vi "LCSS classification.vi"(9 "cluster centers":string[](array[string])=["1 0 -1 1 -1 0 -4 1 -4 0 1", "2 0 -1 2 -1 0 -2 2 -2 0 2", "3 0 -3 3 -3 0 -2 3 -2 0 3", "4 0 -3 4 -3 0 -4 4 -4 0 4", "-1 1 -4 0 -4 4 -3 4 -4 0 -4 1 -1", "-1 2 -2 0 -2 3 -3 3 -2 0 -2 2 -1", "-4 1 -1 0 -1 2 -2 2 -1 0 -1 1 -4", "-4 4 -3 0 -3 3 -2 3 -3 0 -3 4 -4", "0 -4 1 -1 0 -3 3 -2 3 -3 0 -1 1 -4 0", "0 -4 4 -3 0 -1 2 -2 2 -1 0 -3 4 -4 0"], 11 "Patterns in":string[](array[string])=["0 4 0", "4 0 4", "0 4 0", "4 0 4", "0 4 0", "4 0 4", "0 4 0", "4 0 -2", "0 -2 3", "-2 3 0", "3 0 3", "0 3 0", "3 0 4", "0 4 0", "-2 0 1", "0 1 0", "1 0 -4", "0 -4 4", "-2 2 0", "2 0 -1", "0 -1 -4", "-1 -4 1", "-4 1 0", "1 0 3", "0 3 0", "-1 0 -1", "0 -1 2", "0 -1 1", "-1 1 0", "1 0 4", "0 4 0", "4 0 3", "0 3 -2", "3 -2 0", "-2 0 -2", "0 -2 3", "-2 3 -2", "3 -2 0", "-2 0 4", "0 4 0", "4 0 -2", "0 -2 2", "2 -1 0", "-1 0 4", "0 4 0", "4 0 2", "0 2 0", "2 0 -2", "0 -2 0", "1 -1 0", "-1 0 3", "0 3 0", "3 0 -4", "0 -4 4", "-4 4 -4", "4 -4 0", "2 -1 0", "-1 0 3", "0 3 -2", "3 -2 0", "-2 0 -3", "0 -3 0", "-3 0 3", "0 3 0", "3 0 -3", "0 -3 0", "0 4 0", "4 0 4", "0 4 -4", "4 -4 1", "-4 1 -1", "1 -1 0", "-1 0 -3", "0 -3 0", "-3 0 1", "0 1 -4", "1 -4 1", "-4 1 0", "1 0 4", "0 4 0", "4 0 -4", "0 -4 0", "-4 0 -4", "0 -4 4", "-4 4 -4", "4 -4 1", "0 -4 1", "-4 1 0", "1 0 -4", "0 -4 4", "0 4 0", "4 0 -2", "0 -2 2", "-2 2 -2", "2 -2 2", "-2 2 -2", "2 -2 2", "-2 2 -1", "2 -1 0", "-1 0 4", "0 4 0", "4 0 2", "0 2 0", "2 0 4", "0 4 0", "4 0 2", "0 2 -2", "2 -2 0", "-2 0 4", "1 0 -1", "0 -1 0", "-1 0 -1", "0 -1 0", "-1 0 1", "0 1 -1", "-2 2 -2", "2 -2 3", "1 0 -1", "0 -1 0", "-1 0 -1", "0 -1 2", "-1 2 0", "2 0 2", "0 2 -2", "2 -2 0", "-2 0 -4", "0 -4 0", "-2 2 0", "2 0 3", "0 3 -2", "3 -2 2", "1 -1 0", "-1 0 3", "0 4 0", "-2 0 1", "0 1 -4", "1 -4 0", "-4 0 -3", "0 -3 0", "1 0 -1", "0 -1 2", "-1 2 -1", "2 -1 1", "-1 1 -4", "-2 0 -1", "0 -1 1", "0 3 0", "3 0 3", "0 3 0", "3 0 3", "0 3 -2", "-4 0 -4", "0 -4 4", "0 4 0", "4 0 -4", "0 -4 0", "-4 0 -4", "-2 2 0", "2 0 4", "0 4 -4", "4 -4 0", "-4 0 2", "0 2 -2"]) -> (0 "Assigned cluster (0) unassigned":string[](array[string]), 1 "patterns in, distance values":string[][](array[string]), 2 "Assigned cluster 2nd method":string[](array[string]), 3 "Cluster element count":i32[](array[numeric]), 4 "Assigned cluster 3rd method 2":string[](array[string]))   [LabVIEW 2014]
panel:
  in  "Patterns in 2":string[](array[string])
  out "Array":i32[](array[numeric])
  in  "cluster centers 3":string[](array[string])=["0 1 0 -1 1 0 1 -1 0 -4 1 0 1 -4 0", "0 2 0 -1 2 0 2 -1 0 -2 2 0 2 -2 0", "0 3 0 -3 3 0 3 -3 0 -2 3 0 3 -2 0", "0 4 0 -3 4 0 4 -3 0 -4 4 0 4 -4 0", "-1 1 -4 0 -4 4 -3 4 -4 0 -4 1 -1", "-1 2 -2 0 -2 3 -3 3 -2 0 -2 2 -1", "-4 1 -1 0 -1 2 -2 2 -1 0 -1 1 -4", "-4 4 -3 0 -3 3 -2 3 -3 0 -3 4 -4", "0 -4 1 -1 0 -3 3 -2 3 -3 0 -1 1 -4 0", "0 -4 4 -3 0 -1 2 -2 2 -1 0 -3 4 -4 0"]
  out "x .and. y? 2":bool
  out "x .and. y?":bool
  out "number of elements":i32[](array[numeric])
  in  "LEfty CSS":string[](array[string])=["0 4 0", "0 -2 0", "1 -1 0", "-1 2 -1", "0 2 0", "2 -1 0", "0 3 0", "0 -1 0", "-2 0 3", "0 -4 0", "3 -2 0", "0 3 -2", "0 -3 0", "-1 0 3", "0 -2 0 3", "0 1 -1 0", "0 3 -2 0", "1 -4 0", "-1 0 2", "0 -1 2", "2 0 3", "0 -3 3", "3 -3 0", "3 0 -1 0", "-2 0 -2", "2 -2 0", "-3 3 0", "0 2 0 3", "0 1 0", "0 -2 2", "-4 0 -1", "0 -1 2 -1", "-1 0 -1", "2 -1 2", "-1 3 -2", "3 0 -4", "3 -2 2", "-1 1 -1 0", "-1 2 -1 0", "0 1 -4", "4 -4 0", "2 -3 0", "0 3 0 -2", "2 0 3 0", "0 1 0 -3", "1 0 -3", "-1 0 -4 0", "-4 0 1", "2 0 -2 0", "-1 0 -3", "0 -3 4", "4 0 1", "0 1 -4 0", "0 -1 0 3", "0 -3 3 0", "0 3 -3 0", "0 4 0 2", "0 2 -2 0", "-2 0 -3", "3 0 3", "-1 0 -2", "-2 0 3 0", "2 0 4 0", "0 4 0 -2 3", "0 -3 0 -2", "-3 0 -2 2", "1 0 4 0", "-3 0 2", "0 -2 0 3 -2 0", "1 0 -3 0", "-3 0 -2", "-2 0 -2 0", "0 4 -4", "-1 -3 0", "-2 2 -1", "2 0 -3", "-1 1 0", "2 -1 1", "-2 2 0", "0 -4 0 -1", "0 -1 3 -2 2", "-1 2 -1 2", "-1 2 0", "-1 3 0 -1 0", "2 0 2", "-1 0 2 -3 0", "-1 0 2 0", "-1 4 -4 1", "-1 0 4", "2 -1 0 -1", "2 -1 0 2", "-4 1 -1", "3 0 -4 1", "1 -1 -3 3", "0 3 0", "0 2 0", "0 4 0", "0 -3 4", "0 1 0", "2 -1 0", "0 -1 0", "0 -3 3", "2 0 3", "0 4 -4", "1 -1 0", "0 3 -2", "3 0 3", "0 2 -1", "-4 0 -3", "0 -3 0", "-1 0 4", "-1 0 2", "4 -4 1", "4 -4 0", "0 -2 3", "3 -3 0", "0 1 -1", "0 1 -4 0", "3 0 3 0", "1 -4 0", "0 2 0 3", "3 -2 0", "0 3 0 3", "-1 0 3", "1 -1 0 4", "0 2 -1 0", "0 -3 4 -4", "3 0 1", "0 -2 0", "0 4 -4 0", "0 3 0 3 0", "1 0 3 0", "3 -2 2", "-4 0 -3 3", "3 0 -3", "0 -3 3 -3 0", "3 0 -2", "-4 1 0", "0 -4 4", "2 -1 0 -3", "0 3 0 1", "2 0 -3", "-3 0 1", "-4 1 -1", "0 2 -2", "-2 3 0", "1 0 1", "0 -1 0 2", "0 3 -2 2", "0 1 0 3", "0 -4 1", "0 -3 3 0", "-2 2 0", "-2 0 3", "1 0 4 0", "4 -4 1 0", "0 1 -1 2", "1 0 1 0", "0 1 0 1", "-1 0 4 -4", "2 -1 0 3", "1 -1 2", "-1 2 -1 0", "0 4 -4 1 -1", "0 -3 4 -4 1", "4 -4 0 -3 3", "0 -4 4 -4", "-1 0 2 -1", "-2 0 -1", "1 -1 0 4 -4", "0 4 0 3", "2 0 4", "4 -4 0 -3", "0 3 0 -2", "0 -3 4 0", "1 0 3", "-4 0 3", "-3 0 2", "0 3 -2 3", "0 2 0 3 0", "0 4 0 2", "4 -3 0", "-3 0 1 0", "0 2 0 -3", "0 1 0 3 0", "0 -4 0", "0 -4 0 -3", "2 -2 0", "2 0 -2", "0 3 -3", "2 -1 0 -3 4", "-1 0 -2", "1 -1 0 3", "-1 0 3 0", "0 -1 2", "0 -3 4 -4 1 0", "0 4 0 -1", "1 0 -3", "0 3 -2 0", "0 1 0 4 0", "0 4 0 -4", "0 4 0 3 -2", "3 -2 0 1 0", "2 -1 0 -3 0", "-3 0 -4", "0 4 -4 1 -1 0", "-1 0 4 -4 0", "0 4 -4 0 2", "-3 0 -1", "0 3 0 1 -1", "-1 0 4 0", "0 1 -1 2 -1 0", "2 -1 0 2", "0 2 0 -1", "-1 0 -1 0", "-1 0 2 -1 0", "0 1 0 2", "0 2 0 -3 4 -4", "1 0 3 0 2", "0 -2 3 -2", "3 -2 0 -1", "0 4 -4 0 -3", "1 0 -4", "-4 0 -3 3 -3 0", "-2 3 -2 0", "-2 3 -2", "0 4 0 2 0", "-4 0 3 0", "0 1 -4", "0 -3 3 0 -2", "0 -2 0 2", "-2 0 2 0", "3 0 -2 0", "-4 0 -3 0", "0 -3 0 3", "0 3 -3 0", "0 -3 4 -3 0 1 0", "0 3 -2 2 0", "2 0 2", "0 2 0 2 0", "0 3 0 -3", "3 0 -3 4", "0 1 0 1 0", "0 -3 3 -2 0 3", "0 -3 4 -4 0 -3 3 -2", "0 -3 0 2 0", "0 2 -2 0", "0 -3 3 -2", "2 0 -4 0 -3 3", "3 0 -2 3", "0 2 0 -2", "0 2 0 4 0", "-2 0 -2 3 0", "0 1 0 3 0 -2", "-3 3 -3", "0 -3 3 -3", "-3 3 -3 0", "1 0 4", "-4 0 2", "-1 0 -1", "3 0 2", "-3 4 -4", "4 0 3", "-2 0 2", "2 0 3 0", "0 2 -1 0 3", "-3 3 -2", "3 -3 0", "0 3 0", "-3 3 -3 0", "-3 3 -3", "0 -3 3 -3", "0 -3 3 -3 0", "2 -1 0", "0 -3 3", "-3 0 -3", "3 -3 0 -3", "-3 0 -3 3", "0 2 -1", "0 1 0", "0 3 0 3", "0 -1 0", "3 -3 0 -3 3", "0 2 -1 0", "0 4 0", "0 3 -2", "-1 0 2", "3 -2 0", "0 -4 0", "0 -3 0", "3 0 2", "0 3 -3", "0 -3 4", "-3 0 -3 3 -3", "0 3 -2 0", "-1 0 4", "-1 0 3", "-1 0 3 0", "0 1 0 3 0", "1 0 -1", "0 1 0 -1 0", "3 0 1", "0 2 0", "0 -1 2 0", "-3 0 -2", "3 0 -3", "0 -2 3", "0 -3 3 -3 0 -3 3", "3 0 3", "0 2 -1 0 2", "0 2 -2", "2 -2 3", "1 -1 0 3", "0 3 -2 0 1 0", "0 4 0 -1", "0 1 -4", "2 -1 0 4", "0 4 -4", "0 1 0 3 0 1 0", "1 0 3", "0 1 0 3", "1 0 3 0", "2 0 -1", "0 -1 0 3 0 3 0", "0 2 0 3 0", "2 0 4 0 2", "-4 0 -3", "4 -4 0", "0 3 0 3 -3", "-4 0 3 0", "0 -3 4 -3", "-3 3 0", "-2 0 3", "0 -2 0", "1 0 -3", "2 -2 0", "3 0 -3 4", "-3 0 -3 3 -3 0", "3 -3 0 -3 3 -3 0", "0 -3 3 -3 0 -3 3 -3 0", "0 3 0 -3", "-3 3 -3 0 -3", "0 -3 3 -3 0 -3", "-3 3 -3 0 -3 3", "2 -1 0 2", "3 0 3 0", "2 0 3", "3 -3 0 -3 3 -3"]
  in  "Right CSS":string[](array[string])=["0 3 0", "0 1 0", "0 2 0", "0 4 0", "0 4 -4", "0 -3 4", "0 -3 0", "0 -4 0", "0 3 -2", "0 -1 0", "-4 1 0", "1 0 3", "0 2 0 -3", "2 0 3", "3 -3 0", "-3 0 3", "0 -3 3", "0 -3 4 -3 0", "0 -2 0", "3 -2 0", "0 3 0 1 0", "0 -3 4 0", "2 -2 0", "-2 0 -3", "4 0 2", "-3 0 2", "0 3 -3 0", "4 -4 0", "0 -1 2", "3 0 4", "0 3 -2 0", "0 -3 0 3", "1 0 -1", "0 4 -4 0", "-2 0 3", "0 2 -2 0", "0 2 0 -3 4", "3 -3 0 -3", "4 0 2 0", "3 0 -2", "0 -3 3 0", "-1 0 3", "0 -1 2 0", "-4 0 -1", "2 0 3 0", "0 3 0 3", "-4 0 3", "0 4 -4 1", "4 0 -3", "0 -1 0 4", "0 3 -3 0 2", "0 -2 0 3", "0 -3 4 0 3 0", "-3 0 4 0", "0 3 0 3 0", "0 4 0 -3 0", "-3 4 0", "2 0 -3 4", "0 2 0 -3 4 0", "0 1 0 2", "0 -2 3", "-2 0 -2", "0 -3 4 0 2", "0 -3 3 0 -2 2", "1 0 -3", "0 -1 1 0", "4 -4 0 -4", "-4 0 3 0", "2 0 -3", "-2 0 3 0", "0 4 -4 1 0", "-4 1 0 -1 2 0", "3 0 4 -4", "0 -3 4 -3 0 2", "3 0 3", "-1 0 -3", "-3 4 -3", "4 -3 0", "0 -3 4 -3", "-3 4 -3 0", "4 0 2 0 3", "0 2 0 3", "-4 1 0 -4 0 4 -4", "-4 1 -1", "-1 0 -4 0", "1 0 3 -2", "0 -1 0 3", "0 3 0 4 0", "0 2 0 3 0 1 0", "-4 1 -4 1", "1 -4 1 0", "0 -4 4", "0 1 0 4", "1 -4 1", "-3 0 1", "0 4 -4 0 -1 0", "-3 0 4", "2 0 -3 4 0", "1 0 2", "4 -3 0 2", "-3 4 -3 0 2", "3 0 1", "0 3 0", "0 -3 4", "0 -3 3", "0 3 -3 0", "0 2 0", "4 -3 0", "0 3 -3", "0 3 -2", "0 -3 4 -3 0", "-4 0 -3", "3 0 -3", "0 -4 0", "-3 0 -3", "0 -3 3 0 3", "0 -3 3 0", "0 -2 0", "-3 0 3", "3 -3 0", "3 0 3", "-3 4 0", "-4 0 -3 4", "-3 0 4", "0 -1 0", "3 0 -3 3", "-3 3 0", "0 3 -2 0", "0 -3 4 0", "1 0 -3 4", "0 -3 0", "0 -1 0 -3", "-3 0 3 0", "-2 0 3 -2", "0 1 0", "0 -2 0 3", "-2 0 -3", "0 3 0 -3", "3 0 3 -3", "3 -3 0 3", "-3 0 -3 3 0", "0 -3 4 -4 0", "0 2 0 -2", "-2 0 3", "0 3 -2 3 0", "-2 3 0 -3 3", "3 0 -1", "-3 0 -4", "1 -1 0", "-4 0 -2", "0 3 -3 0 4", "-2 3 0", "-1 0 3 -2", "-3 4 -3", "0 -3 4 -3", "-3 4 -3 0", "-3 3 0 3", "-2 0 2", "0 3 0", "0 -1 0", "0 4 0", "-1 0 3", "0 -3 4", "0 -3 3", "1 -1 0", "0 3 -2", "0 2 0", "0 1 -1", "4 -3 0", "-4 0 -3", "0 -4 0", "4 0 2", "0 1 -1 0", "0 1 0", "0 4 -4", "3 -2 2", "2 -1 0", "0 -2 0", "0 -3 4 0", "-1 0 -3", "0 3 -2 0", "0 -3 3 -3 0", "0 -3 4 -3 0", "4 0 4", "0 1 -1 0 3", "3 -2 2 0", "-2 2 0", "3 0 1", "0 4 0 2", "0 2 -1", "2 0 4", "-1 0 4", "0 -3 3 0", "-1 0 1", "-1 0 -1 0", "-1 0 -1", "4 -3 0 2", "0 -3 0", "-4 0 -3 0", "-3 0 3 -2", "0 3 -2 2 0", "-4 0 -3 3", "0 3 0 -4", "2 0 4 -4", "0 2 0 4", "0 4 0 -4", "2 -1 0 1 -1 0", "0 2 -1 0", "-1 0 -3 3", "0 -4 4 0", "0 4 -4 0", "-4 0 3 0", "0 -2 3", "-3 0 -3", "0 -2 0 -3", "-3 0 1", "-2 3 0", "0 3 0 -2", "0 4 -3 0", "4 -3 0 2 0", "0 -3 4 -3 0 3 -2 2 0", "3 0 -3 4 -3 0", "-1 0 3 -2 3", "-1 0 3 -2", "0 1 0 3", "1 0 3", "4 -3 0 -2", "-4 0 -3 4", "-2 0 3 0", "2 0 2", "0 2 0 2 0", "-4 4 -3 0", "0 -4 0 -3", "3 0 3 0", "-4 0 -3 3 0", "4 0 3", "0 4 0 4", "4 0 4 0", "0 4 0 -4 0", "0 -1 0 -2", "4 0 2 0", "1 0 -3", "0 -4 1 -4", "0 4 -4 0 -3", "-2 2 0 4 -4", "0 4 -4 4 -4", "4 0 2 -2", "0 4 0 -2", "0 3 0 1", "4 -4 1", "4 0 2 -1 0", "0 -4 4 0 2", "-1 0 3 0", "0 3 -2 0 -1 0", "1 -1 0 4", "0 4 0 1", "-1 0 4 0", "1 0 3 -2 0 -1 0", "0 -4 0 3 0 -4", "-1 0 -4", "1 -4 0", "1 0 4 0", "0 -1 0 -1 0", "-1 0 -3 3 0", "0 -1 0 -1 0 -3", "-2 2 -1 0", "0 -1 0 3 -2", "2 -1 0 1 -1 0 3", "-2 3 -2 2 -1", "-2 2 -1", "0 -1 0 4", "3 0 1 0", "0 3 -2 0 -1 0 -1 0", "-3 4 0", "3 0 -1", "0 4 -3", "3 0 3", "-4 0 3", "4 -4 0", "0 -1 0 -1", "1 -1 0", "0 -1 0", "0 1 0", "0 1 -1 0", "0 4 0", "0 3 0", "-1 0 4", "-1 0 -3 3", "1 0 1", "-4 1 -1", "0 4 0 2", "0 -1 0 -3", "3 -2 2 -1 0", "2 -1 0", "0 1 -1", "-1 0 3", "-1 1 -1 0", "-3 0 1", "-1 0 3 0 -4", "-1 0 -3", "1 -1 0 -3 3", "1 -1 0 3", "2 -1 0 4 -4", "1 0 1 0", "0 -1 0 4", "2 0 3 0 -1", "-4 1 -1 0", "0 4 0", "0 3 0", "0 2 0", "4 -4 0", "0 4 -4 0", "0 -2 0", "3 -3 0", "0 4 -4", "0 3 -3", "0 3 -2", "0 4 0 2", "4 0 2", "0 1 0", "0 3 -3 0", "0 -3 0", "2 -1 0", "0 -1 0", "1 0 3", "4 0 3", "3 -2 0", "0 1 -4", "-1 0 4", "0 -4 0", "0 -3 3", "2 0 4", "-4 1 0", "0 -2 2", "0 4 0 3", "-1 0 1", "0 3 -2 0", "-3 0 4", "-1 0 3", "0 -3 4", "0 4 0 -2", "1 -1 0", "2 0 4 0", "0 -4 4", "0 -1 0 4", "-1 0 4 0", "4 -3 0", "0 2 -1 0", "1 -4 0", "2 0 -4", "-2 0 4", "0 4 0 2 0", "3 0 3", "0 -3 3 0", "2 -2 0", "1 0 -3", "-4 0 2", "1 0 3 0", "0 1 0 3", "-1 0 3 0", "3 -2 2", "-4 1 -1", "2 0 -3", "0 -4 1", "0 2 0 -4", "-3 0 4 0", "3 0 -2", "0 -2 2 0", "0 -2 3", "-4 0 2 0", "0 3 0 -4", "0 2 0 4 0", "-2 0 2", "-2 2 0", "0 3 0 4", "-3 4 0", "-1 0 1 0", "4 0 4", "0 1 0 3 0", "0 -1 0 4 0", "0 3 0 3", "1 0 -3 0", "0 3 0 1", "-2 2 -1 0", "0 3 -2 2", "-3 0 2", "1 -1 0 3 0", "0 3 0 -2", "-4 0 -4", "0 1 0 -3 0", "0 4 0 -3", "2 -1 0 4", "1 -4 1", "-4 0 3", "-2 0 -4 0", "0 3 -3 0 4", "-4 0 -2", "0 4 -4 0 3", "0 -2 3 -2 0", "0 4 0 4", "-1 2 -1", "-3 0 -2", "-3 0 -3", "-4 0 4", "4 0 -3", "3 0 -4", "2 0 -2", "-2 0 2 0", "0 -4 4 0", "0 2 0 3", "-2 0 1", "4 0 3 -3 0", "0 -2 0 3", "0 4 0 3 0", "0 2 -2 0", "2 -2 0 4", "4 0 -2", "2 0 -1", "0 1 -4 0", "0 -1 2", "4 0 -1", "0 1 -4 1", "4 -4 1", "0 3 -2 0 1", "4 0 4 0", "0 -1 0 4 0 4", "1 0 4", "0 1 -4 1 0", "0 4 0 2 0 -3", "-2 0 4 0", "0 2 -2 0 4 0", "0 -3 0 2", "-4 0 -2 0", "0 -2 0 2 0", "0 2 0 -1", "0 -1 3", "0 -4 4 -4", "3 -2 0 -4 0", "-4 0 -1", "-3 0 3 0 3", "-1 0 3 -3 0", "-3 0 3 0", "0 3 0 3 -2", "-2 2 -2", "-1 0 1 0 3", "-2 2 -1 0 1 0", "0 2 -1 0 -3", "0 4 0 2 -1 0", "-1 0 4 -4 0", "0 2 -1 0 4 -4", "0 4 -4 0 3 -2 0", "-1 0 -3", "-2 0 1 -4", "0 3 0 4 0", "0 1 -4 4", "-1 0 -3 0", "-1 0 4 -4", "0 4 0 -2 0", "0 4 -3 0", "4 0 -3 3", "-1 0 -2", "0 -2 0 3 -3", "1 -4 1 -1 0", "-4 1 -1 0", "-2 0 -2 2", "0 -1 2 -1", "-4 0 -4 1", "0 2 0 4 0 2 0", "0 3 0 -1", "3 0 3 0", "0 -3 0 3 0", "0 3 0 4 -4 1", "-1 0 -4", "0 -4 1 0 3 0", "0 2 -1", "-4 0 4 0", "0 -2 0 4", "0 4 0 -1", "-4 0 3 0", "0 3 0 -2 0", "0 -3 4 -3 0", "-4 0 2 0 -4", "2 0 -2 0", "-2 2 0 -3", "3 0 2 0 4 0", "3 0 2 0", "1 -4 0 2 0", "3 0 -4 4 0", "3 0 -4 4", "3 -3 0 4", "-2 3 -3", "0 -4 0 2 0", "0 3 0 -4 0", "3 -3 0 4 0", "0 3 -3 0 4 0", "4 0 3 -2", "-4 0 -3", "-3 0 -3 4", "3 -3 4 0", "1 -4 -1", "-3 3 -3 0", "0 -1 1", "-3 0 4 0 3", "0 3 -3 0 -2", "0 4 0 3 -3 0", "4 -3 0 4", "0 3 0 2 0", "0 4 0 -2 2", "-4 -1 0 1", "-1 0 1 0 -3 0", "-3 0 1 -4 0", "-3 3 0", "0 -1 0 1", "-1 0 1 -4", "0 3 0 -4 4", "-4 1 -1 0 3 0", "0 1 0 3 0 1", "-3 0 3", "4 0 -2 0", "4 0 2 0", "3 0 -1", "4 0 3 -3", "3 -3 0 -2", "3 0 4", "3 0 2", "2 0 3", "4 0 -2 2", "-2 2 -1", "0 4 0", "0 2 0", "0 3 0", "0 -3 0", "0 1 0", "-4 0 -3", "0 -4 0", "0 3 -3 0", "0 -3 0 3", "-4 0 3", "0 4 0 2", "0 -3 3", "-4 0 -3 0 3", "0 2 0 3", "-3 0 2", "0 4 0 1", "0 -4 0 3", "0 4 0 2 0", "0 -2 0", "0 1 0 4", "4 0 2", "0 1 0", "0 -1 0", "0 2 0", "0 4 0", "-4 1 0", "0 -4 0", "0 -2 0", "1 0 4", "1 -4 0", "0 -3 3", "0 -3 0", "1 -1 0", "-2 2 0", "0 1 -4", "2 0 -3", "0 -3 3 0", "-1 0 -1", "0 -1 1", "2 -1 0", "0 2 -1", "-3 0 1", "0 1 0 4", "1 0 4 0", "-3 3 0", "1 0 -3", "3 -2 0", "2 0 -3 0", "1 0 -1", "-4 0 -1", "0 -4 1", "2 0 -1", "0 -2 2", "-4 0 -3", "0 -1 1 0", "0 2 0 -3", "3 -3 0", "-4 0 1 0", "-4 1 -4 0", "-4 1 0 4", "0 1 -4 0", "-4 1 -4", "0 2 -1 0", "1 0 3", "0 -3 4 0", "-2 0 2", "1 0 1", "4 0 2 0", "0 2 0 3", "0 -1 2", "-1 0 -4", "1 0 -4", "0 -1 0 -1", "-1 0 2", "-1 0 -1 0", "1 0 -2", "0 -4 0 -1", "0 -2 2 0", "-1 0 1", "2 0 2", "0 1 -1 0", "0 3 -3 0", "-4 0 -2", "0 4 -4", "0 -4 0 -3", "0 4 0 1", "0 -2 0 2", "0 4 0 2 0", "-3 0 1 -4 0 -3", "2 0 1 0", "-2 0 2 0", "0 3 -2 0", "-3 3 0 -2 0", "3 -3 0 1", "-3 0 1 0", "4 -4 0", "0 4 -4 0", "0 -3 3 0 -2", "2 0 2 0", "-2 0 -1", "0 -4 0 1 0", "2 0 -4 0", "2 0 -1 0", "-1 3 -2", "2 0 1", "1 0 -3 3 0", "-4 1 -1", "-4 1 -1 0", "-1 0 -3", "3 -2 2", "-1 1 -1 0", "2 0 4", "1 0 -1 0", "0 -1 2 -1", "0 2 0 -2", "-3 0 -4 1", "0 1 0 -1", "-1 3 0", "0 -1 0 -4", "-2 0 -1 0", "4 0 4", "-4 1 0 4 0", "-4 0 -2 0", "-4 0 2", "0 -2 0 2 0", "0 2 0 -4 0", "2 0 4 0", "4 0 -2", "0 1 0 -4 0", "3 0 1", "2 -2 0", "4 0 -2 0", "0 2 0 4", "1 -4 0 1 0", "0 2 0 -2 0", "-2 2 0 -1 0", "-2 2 0 -1", "-1 0 4 0", "-2 0 4", "-4 1 0 3", "0 -3 0 1", "-2 2 0 -3 0", "0 1 0 3", "0 2 0 1", "0 1 0 1 -4", "0 1 -4 1", "-4 1 0 -3", "1 0 -3 0", "-3 0 -2", "2 -1 0 -1 0", "-3 3 0 -2", "1 0 4 -4 0", "0 -4 0 -3 0", "0 -4 0 1 0 -3 3 0", "0 -3 3 0 2 0 -3 0", "0 -3 3 -3 0", "3 -2 0 1", "-4 0 3", "-2 0 1", "0 3 0", "0 -3 4", "-3 4 0", "-3 0 4", "0 3 -3 0 1 -4 0 -3 3", "0 -2 0 -1", "-4 1 0 -2", "-4 0 -2 0 -1", "-2 0 -4", "0 1 0 -2", "0 -1 0 2 0", "0 -2 2 0 -1", "0 -3 -1 3", "-4 -1 0", "0 -1 2 0", "0 -3 0 -4", "2 0 -3 0 -4", "3 0 -1 1", "-4 1 0 -1", "-1 0 -1 2", "-1 0 -4 0", "0 -4 1 -1", "-3 3 -2", "2 -1 1", "4 -3 0", "1 -4 4", "0 2 0 -1", "1 0 1 0", "4 1 0", "0 2 0 2 0", "-4 0 -1 -3", "1 -4 0 -1", "0 -4 1 -4", "-1 3 0 -4 1 -4", "2 -1 3", "1 -3 0", "-2 0 1 -4", "1 0 -1 1", "0 -3 0 -4 1", "0 2 -1 0 1 -4", "0 -1 3", "0 -4 0 -1 0", "0 4 0 -2", "0 -2 0 -1 0", "0 -3 3 0 -2 0", "0 1 -1 0 -1", "0 -1 0 1 -1 0", "-1 3 -2 2", "-2 2 0 1 0 -1", "0 1 -1", "0 4 0 1 0 4", "-3 0 -4", "1 0 4 0 4 0", "4 -4 0 -2", "4 0 2", "-1 2 0", "1 -1 0 -1", "4 0 1", "2 0 3"]
  in  "Jon CSS only":string[](array[string])=["0 3 0", "0 1 0", "0 2 0", "0 4 0", "0 4 -4", "0 -3 4", "0 -3 0", "0 -4 0", "0 3 -2", "0 -1 0", "-4 1 0", "1 0 3", "0 2 0 -3", "2 0 3", "3 -3 0", "-3 0 3", "0 -3 3", "0 -3 4 -3 0", "0 -2 0", "3 -2 0", "0 3 0 1 0", "0 -3 4 0", "2 -2 0", "-2 0 -3", "4 0 2", "-3 0 2", "0 3 -3 0", "4 -4 0", "0 -1 2", "3 0 4", "0 3 -2 0", "0 -3 0 3", "1 0 -1", "0 4 -4 0", "-2 0 3", "0 2 -2 0", "0 2 0 -3 4", "3 -3 0 -3", "4 0 2 0", "3 0 -2", "0 -3 3 0", "-1 0 3", "0 -1 2 0", "-4 0 -1", "2 0 3 0", "0 3 0 3", "-4 0 3", "0 4 -4 1", "4 0 -3", "0 -1 0 4", "0 3 -3 0 2", "0 -2 0 3", "0 -3 4 0 3 0", "-3 0 4 0", "0 3 0 3 0", "0 4 0 -3 0", "-3 4 0", "2 0 -3 4", "0 2 0 -3 4 0", "0 1 0 2", "0 -2 3", "-2 0 -2", "0 -3 4 0 2", "0 -3 3 0 -2 2", "1 0 -3", "0 -1 1 0", "4 -4 0 -4", "-4 0 3 0", "2 0 -3", "-2 0 3 0", "0 4 -4 1 0", "-4 1 0 -1 2 0", "3 0 4 -4", "0 -3 4 -3 0 2", "3 0 3", "-1 0 -3", "-3 4 -3", "4 -3 0", "0 -3 4 -3", "-3 4 -3 0", "4 0 2 0 3", "0 2 0 3", "-4 1 0 -4 0 4 -4", "-4 1 -1", "-1 0 -4 0", "1 0 3 -2", "0 -1 0 3", "0 3 0 4 0", "0 2 0 3 0 1 0", "-4 1 -4 1", "1 -4 1 0", "0 -4 4", "0 1 0 4", "1 -4 1", "-3 0 1", "0 4 -4 0 -1 0", "-3 0 4", "2 0 -3 4 0", "1 0 2", "4 -3 0 2", "-3 4 -3 0 2", "3 0 1", "0 3 0", "0 -3 4", "0 -3 3", "0 3 -3 0", "0 2 0", "4 -3 0", "0 3 -3", "0 3 -2", "0 -3 4 -3 0", "-4 0 -3", "3 0 -3", "0 -4 0", "-3 0 -3", "0 -3 3 0 3", "0 -3 3 0", "0 -2 0", "-3 0 3", "3 -3 0", "3 0 3", "-3 4 0", "-4 0 -3 4", "-3 0 4", "0 -1 0", "3 0 -3 3", "-3 3 0", "0 3 -2 0", "0 -3 4 0", "1 0 -3 4", "0 -3 0", "0 -1 0 -3", "-3 0 3 0", "-2 0 3 -2", "0 1 0", "0 -2 0 3", "-2 0 -3", "0 3 0 -3", "3 0 3 -3", "3 -3 0 3", "-3 0 -3 3 0", "0 -3 4 -4 0", "0 2 0 -2", "-2 0 3", "0 3 -2 3 0", "-2 3 0 -3 3", "3 0 -1", "-3 0 -4", "1 -1 0", "-4 0 -2", "0 3 -3 0 4", "-2 3 0", "-1 0 3 -2", "-3 4 -3", "0 -3 4 -3", "-3 4 -3 0", "-3 3 0 3", "-2 0 2", "0 3 0", "0 -1 0", "0 4 0", "-1 0 3", "0 -3 4", "0 -3 3", "1 -1 0", "0 3 -2", "0 2 0", "0 1 -1", "4 -3 0", "-4 0 -3", "0 -4 0", "4 0 2", "0 1 -1 0", "0 1 0", "0 4 -4", "3 -2 2", "2 -1 0", "0 -2 0", "0 -3 4 0", "-1 0 -3", "0 3 -2 0", "0 -3 3 -3 0", "0 -3 4 -3 0", "4 0 4", "0 1 -1 0 3", "3 -2 2 0", "-2 2 0", "3 0 1", "0 4 0 2", "0 2 -1", "2 0 4", "-1 0 4", "0 -3 3 0", "-1 0 1", "-1 0 -1 0", "-1 0 -1", "4 -3 0 2", "0 -3 0", "-4 0 -3 0", "-3 0 3 -2", "0 3 -2 2 0", "-4 0 -3 3", "0 3 0 -4", "2 0 4 -4", "0 2 0 4", "0 4 0 -4", "2 -1 0 1 -1 0", "0 2 -1 0", "-1 0 -3 3", "0 -4 4 0", "0 4 -4 0", "-4 0 3 0", "0 -2 3", "-3 0 -3", "0 -2 0 -3", "-3 0 1", "-2 3 0", "0 3 0 -2", "0 4 -3 0", "4 -3 0 2 0", "0 -3 4 -3 0 3 -2 2 0", "3 0 -3 4 -3 0", "-1 0 3 -2 3", "-1 0 3 -2", "0 1 0 3", "1 0 3", "4 -3 0 -2", "-4 0 -3 4", "-2 0 3 0", "2 0 2", "0 2 0 2 0", "-4 4 -3 0", "0 -4 0 -3", "3 0 3 0", "-4 0 -3 3 0", "4 0 3", "0 4 0 4", "4 0 4 0", "0 4 0 -4 0", "0 -1 0 -2", "4 0 2 0", "1 0 -3", "0 -4 1 -4", "0 4 -4 0 -3", "-2 2 0 4 -4", "0 4 -4 4 -4", "4 0 2 -2", "0 4 0 -2", "0 3 0 1", "4 -4 1", "4 0 2 -1 0", "0 -4 4 0 2", "-1 0 3 0", "0 3 -2 0 -1 0", "1 -1 0 4", "0 4 0 1", "-1 0 4 0", "1 0 3 -2 0 -1 0", "0 -4 0 3 0 -4", "-1 0 -4", "1 -4 0", "1 0 4 0", "0 -1 0 -1 0", "-1 0 -3 3 0", "0 -1 0 -1 0 -3", "-2 2 -1 0", "0 -1 0 3 -2", "2 -1 0 1 -1 0 3", "-2 3 -2 2 -1", "-2 2 -1", "0 -1 0 4", "3 0 1 0", "0 3 -2 0 -1 0 -1 0", "-3 4 0", "3 0 -1", "0 4 -3", "3 0 3", "-4 0 3", "4 -4 0", "0 -1 0 -1", "1 -1 0", "0 -1 0", "0 1 0", "0 1 -1 0", "0 4 0", "0 3 0", "-1 0 4", "-1 0 -3 3", "1 0 1", "-4 1 -1", "0 4 0 2", "0 -1 0 -3", "3 -2 2 -1 0", "2 -1 0", "0 1 -1", "-1 0 3", "-1 1 -1 0", "-3 0 1", "-1 0 3 0 -4", "-1 0 -3", "1 -1 0 -3 3", "1 -1 0 3", "2 -1 0 4 -4", "1 0 1 0", "0 -1 0 4", "2 0 3 0 -1", "-4 1 -1 0"]
  out "transposed array":dbl[][](array[numeric])
  out "appended array":string[][](array[string])
  out "Distance values (LCS)":dbl[][](array[numeric])
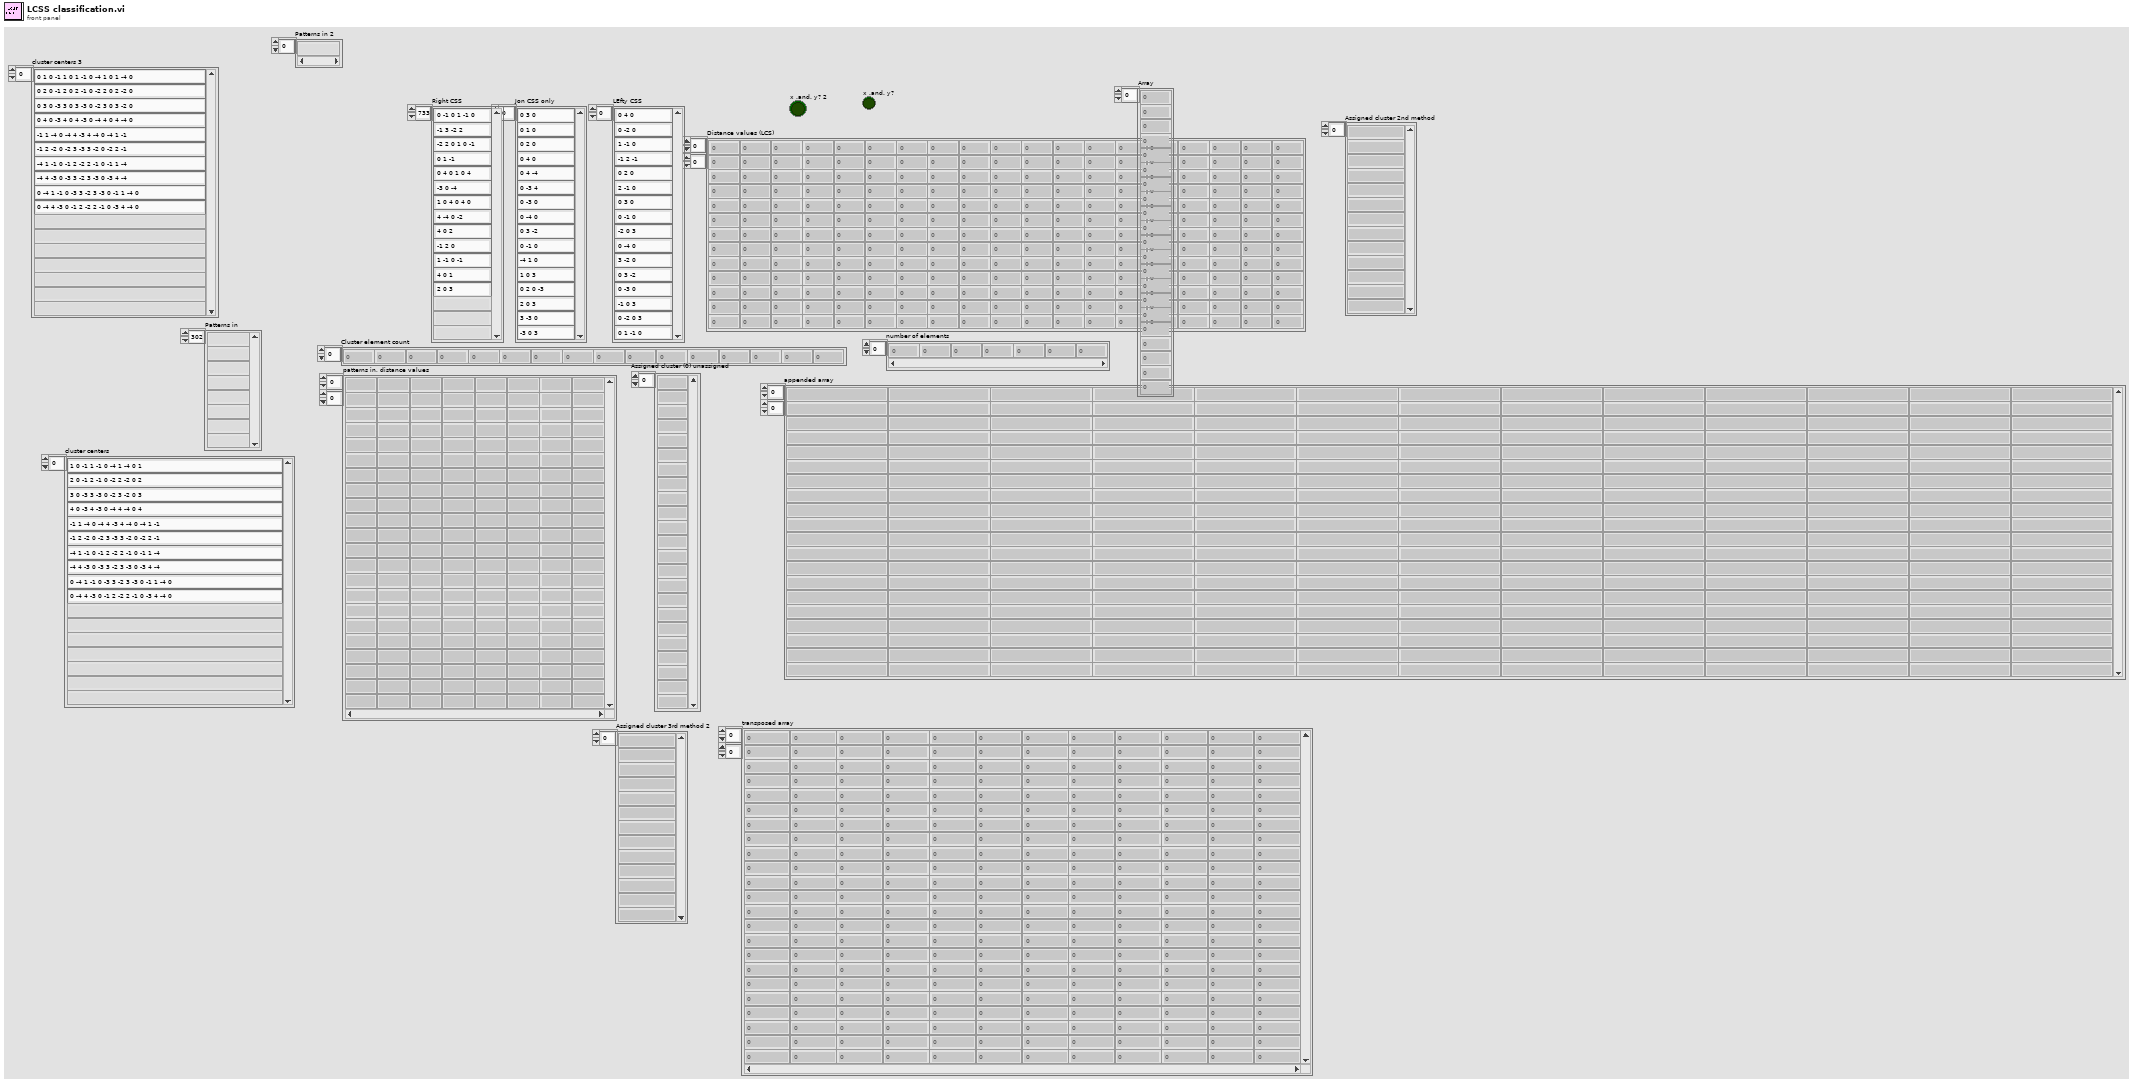
[diagram p1: front panel]
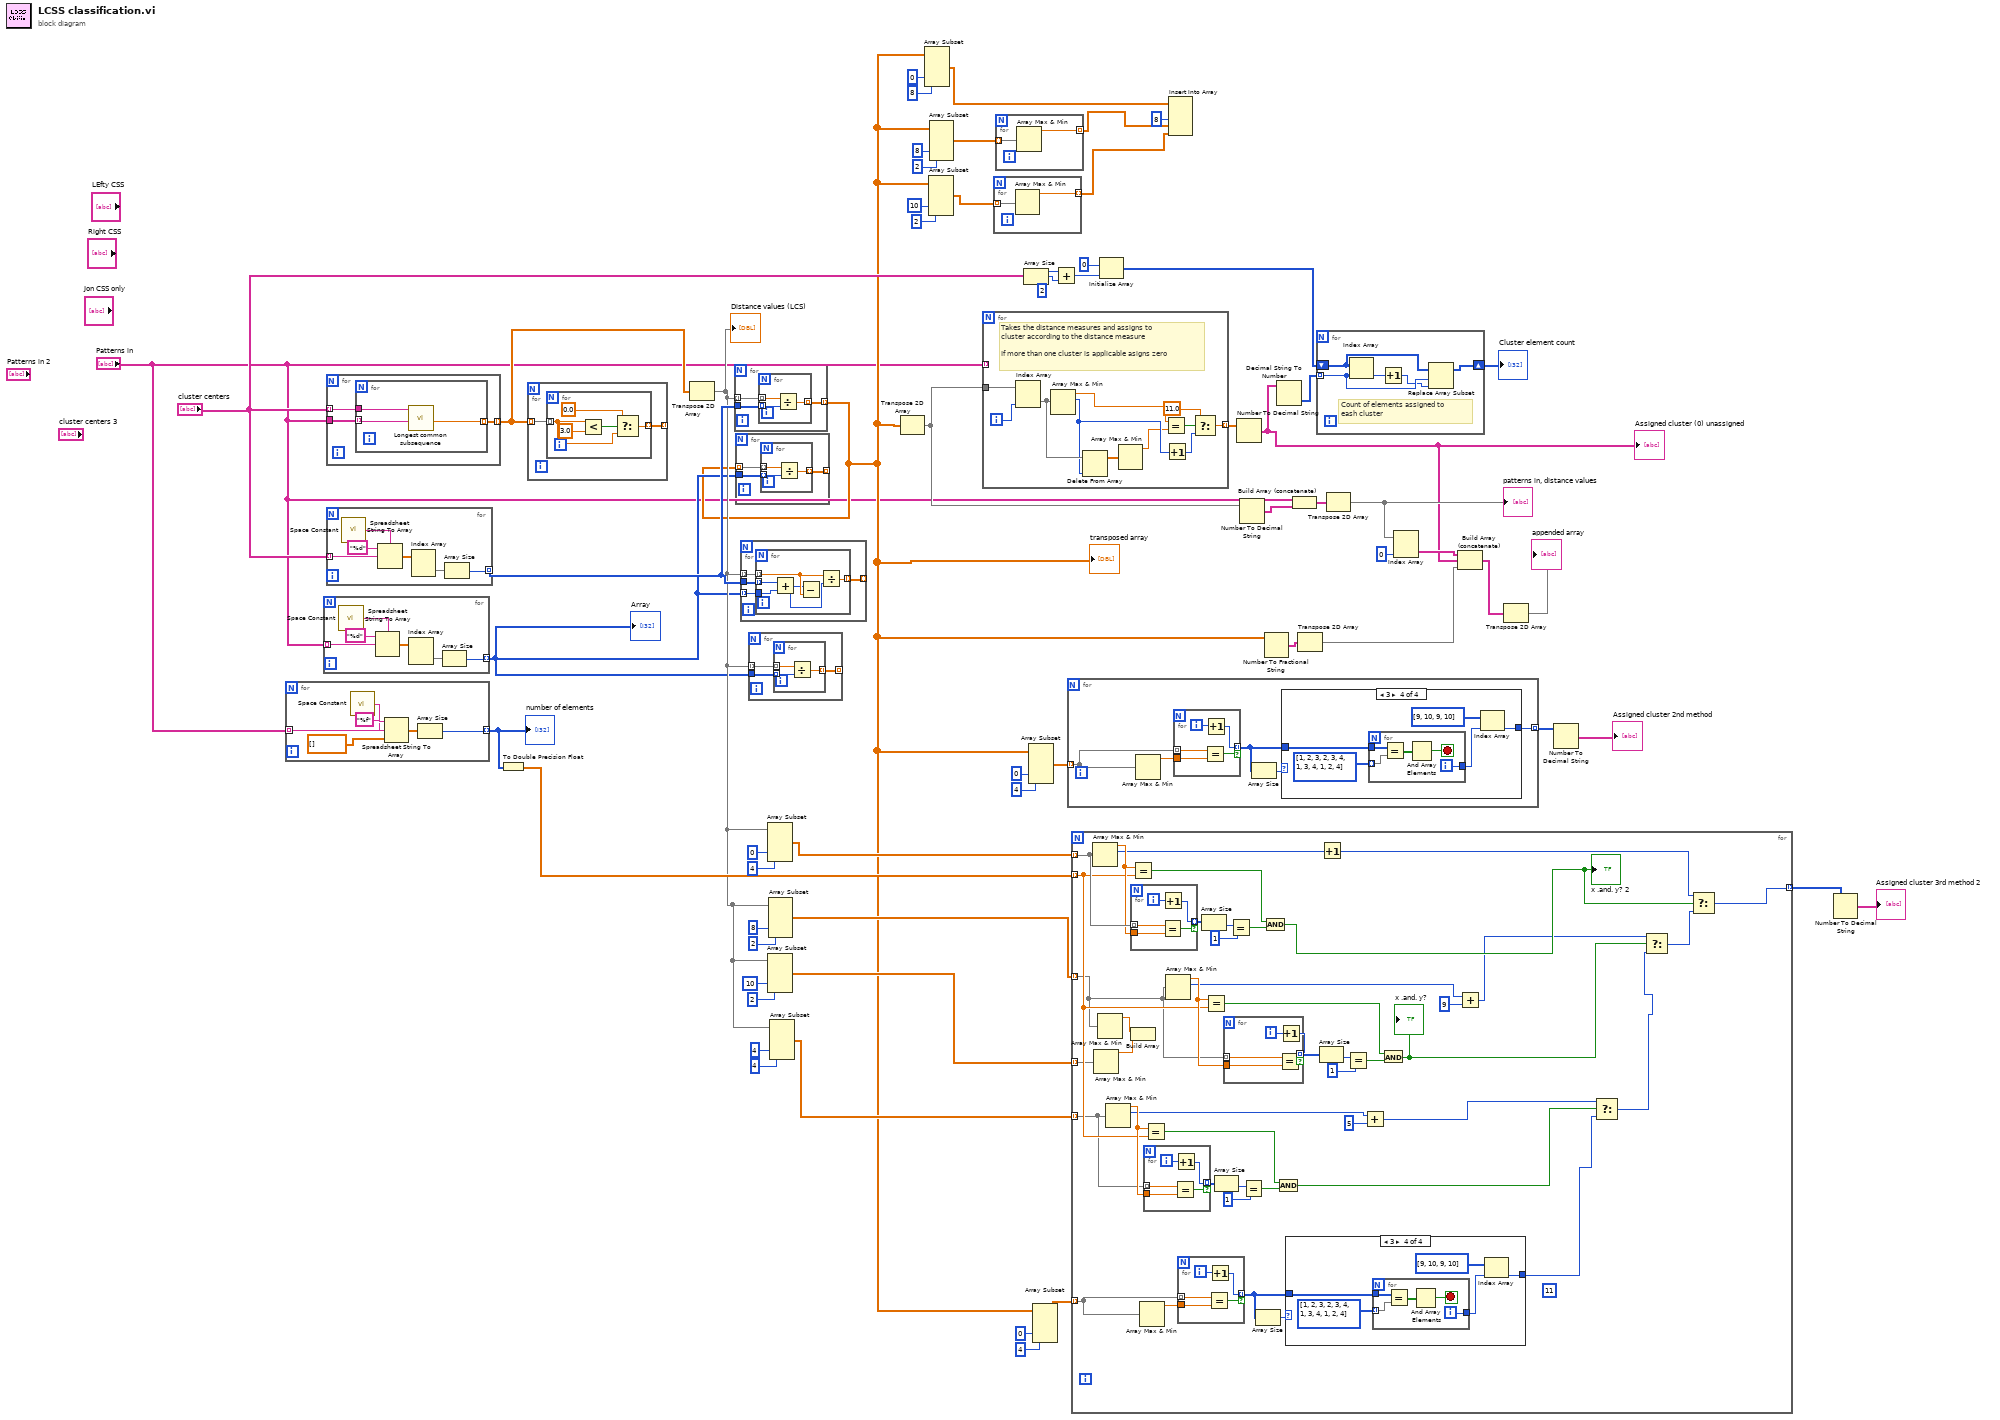
[diagram p0: block diagram]
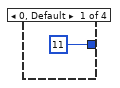
[diagram p2: hidden frame]
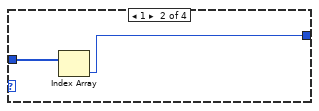
[diagram p3: hidden frame]
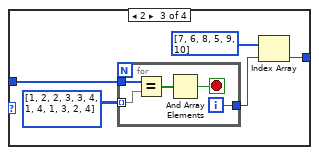
[diagram p4: hidden frame]
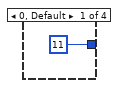
[diagram p5: hidden frame]
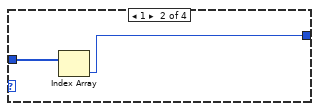
[diagram p6: hidden frame]
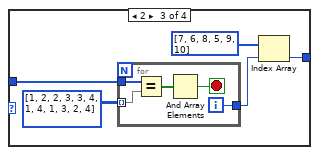
[diagram p7: hidden frame]
diagram:
  n1 = for {
    tunnel: "Patterns in" -> [w65] mode=indexing
    tunnel: [w63] -> w31 mode=indexing
    n2 = call <vilib>:"Space Constant.vi"() -> ("String"=w67:string)
    n3 = Spreadsheet String To Array(delimiter (Tab)=w67, format string="%f", spreadsheet string=w65, array type (2D Dbl)=dbl[] [] ("array 2")) -> (array=w64:dbl[])
    n4 = Array Size(array=w64) -> (size(s)=w63:i32)
  }
  "number of elements" <- w31
  n5 = for {
    tunnel: "Patterns in" -> [w73] mode=indexing
    tunnel: [w69] -> w4 mode=indexing
    n6 = call <vilib>:"Space Constant.vi"() -> ("String"=w74:string)
    n7 = Spreadsheet String To Array(delimiter (Tab)=w74, format string="%d", spreadsheet string=w73) -> (array=w71:dbl[][])  [unwired: 1 in]
    n8 = Index Array(array=w71) -> (element=w70:dbl[])  [unwired: 2 in]
    n9 = Array Size(array=w70) -> (size(s)=w69:i32)
  }
  "Array" <- w4
  n10 = for {
    tunnel: "cluster centers" -> [w77] mode=indexing
    tunnel: [w76] -> w44 mode=indexing
    tunnel: "Patterns in" -> [w75]
    n11 = for {
      tunnel: w75 -> [w79] mode=indexing
      tunnel: w77 -> [w80]
      tunnel: [w78] -> w76 mode=indexing
      n12 = call "Longest common subsequence.vi"("Pattern 2 COLUMN(0)"=w79, "Pattern 1 ROW(0)"=w80) -> ("LCS length"=w78:dbl)  [unwired: 8 in, 1 out]
    }
  }
  n13 = for {
    tunnel: "cluster centers" -> [w85] mode=indexing
    tunnel: [w81] -> w6 mode=indexing
    n14 = call <vilib>:"Space Constant.vi"() -> ("String"=w86:string)
    n15 = Spreadsheet String To Array(delimiter (Tab)=w86, format string="%d", spreadsheet string=w85) -> (array=w83:dbl[][])  [unwired: 1 in]
    n16 = Index Array(array=w83) -> (element=w82:dbl[])  [unwired: 2 in]
    n17 = Array Size(array=w82) -> (size(s)=w81:i32)
  }
  n18 = To Double Precision Float(number=w31) -> (double precision float=w30:dbl[])
  n19 = for {
    tunnel: w44 -> [w88] mode=indexing
    tunnel: [w87] -> _ mode=indexing
    n20 = for {
      tunnel: w88 -> [w90] mode=indexing
      tunnel: [w89] -> w87 mode=indexing
      n21 = Less?(x=w90, y=3.0) -> (x < y?=w92:bool)
      n22 = Select(t=0.0, s=w92, f=w90) -> (s? t:f=w89:dbl)
    }
  }
  n23 = Transpose 2D Array(2D array=w44) -> (transposed array=w5:dbl[][])
  "Distance values (LCS)" <- w5
  n24 = for {
    tunnel: w5 -> [w96] mode=indexing
    tunnel: w6 -> [w95]
    tunnel: [w94] -> w2 mode=indexing
    n25 = for {
      tunnel: w96 -> [w99] mode=indexing
      tunnel: w95 -> [w98] mode=indexing
      tunnel: [w97] -> w94 mode=indexing
      n26 = Divide(x=w99, y=w98) -> (x/y=w97:dbl)
    }
  }
  "transposed array" <- w2
  n27 = for {
    tunnel: w2 -> [w102] mode=indexing
    tunnel: w4 -> [w101]
    tunnel: [w100] -> _ mode=indexing
    n28 = for {
      tunnel: w102 -> [w105] mode=indexing
      tunnel: w101 -> [w104] mode=indexing
      tunnel: [w103] -> w100 mode=indexing
      n29 = Divide(x=w105, y=w104) -> (x/y=w103:dbl)
    }
  }
  n30 = for {
    tunnel: w5 -> [w109] mode=indexing
    tunnel: w6 -> [w108]
    tunnel: [w107] -> _ mode=indexing
    tunnel: w4 -> [w106] mode=indexing
    n31 = for {
      tunnel: w109 -> [w112] mode=indexing
      tunnel: w108 -> [w113] mode=indexing
      tunnel: [w114] -> w107 mode=indexing
      tunnel: w106 -> [w111]
      n32 = Add(x=w113, y=w111) -> (x+y=w110:i32)
      n33 = Subtract(x=w110, y=w112) -> ()  [unwired: 1 out]
      n34 = Divide(x=w112, y=w110) -> (x/y=w114:dbl)
    }
  }
  n35 = for {
    tunnel: w5 -> [w117] mode=indexing
    tunnel: w4 -> [w116]
    tunnel: [w115] -> _ mode=indexing
    n36 = for {
      tunnel: w117 -> [w120] mode=indexing
      tunnel: w116 -> [w119] mode=indexing
      tunnel: [w118] -> w115 mode=indexing
      n37 = Divide(x=w120, y=w119) -> (x/y=w118:dbl)
    }
  }
  n38 = Array Subset(array=w5, index (col)=0 ("index"), length (col)=4 ("length")) -> (w32:dbl[][])  [unwired: 2 in]
  n39 = Array Subset(array=w5, index (col)=10 ("index"), length (col)=2 ("length")) -> (w19:dbl[][])  [unwired: 2 in]
  n40 = Array Subset(array=w5, index (col)=8 ("index"), length (col)=2 ("length")) -> (w28:dbl[][])  [unwired: 2 in]
  n41 = Array Subset(array=w5, index (col)=4 ("index"), length (col)=4 ("length")) -> (w23:dbl[][])  [unwired: 2 in]
  n42 = Transpose 2D Array(2D array=w2) -> (transposed array=w46:dbl[][])
  n43 = Array Subset(array=w2, index (col)=0 ("index"), length (col)=8 ("length")) -> (w10:dbl[][])  [unwired: 2 in]
  n44 = Array Subset(array=w2, index (col)=10 ("index"), length (col)=2 ("length")) -> (w11:dbl[][])  [unwired: 2 in]
  n45 = Array Subset(array=w2, index (col)=8 ("index"), length (col)=2 ("length")) -> (w12:dbl[][])  [unwired: 2 in]
  n46 = for {
    tunnel: "Patterns in" -> [_] mode=indexing
    tunnel: w46 -> [w131]
    tunnel: [w121] -> w62 mode=indexing
    i -> [w130]
    # "Takes the distance measures and assigns to \ncluster according to the distance measure\n\nIf more than one cluster is applicable asigns zero"
    n47 = Index Array(array=w131, index (col)=w130) -> (element=w125:dbl[])  [unwired: 1 in]
    n48 = Array Max & Min(array=w125) -> (max value=w124:dbl, max index (indices)=w123:i32)  [unwired: 2 out]
    n49 = Delete From Array(array=w125, index=w123) -> (array with subset deleted=w129:dbl[])  [unwired: 1 in, 1 out]
    n50 = Array Max & Min(array=w129) -> (max value=w122:dbl)  [unwired: 3 out]
    n51 = Equal?(x=w124, y=w122) -> (x = y?=w128:bool)
    n52 = Increment(x=w123) -> (x+1=w126:i32)
    n53 = Select(t=11.0, s=w128, f=w126) -> (s? t:f=w121:dbl)
  }
  n54 = for {
    tunnel: w11 -> [w133] mode=indexing
    tunnel: [w132] -> w8 mode=indexing
    n55 = Array Max & Min(array=w133) -> (max value=w132:dbl)  [unwired: 3 out]
  }
  n56 = for {
    tunnel: w12 -> [w135] mode=indexing
    tunnel: [w134] -> w9 mode=indexing
    n57 = Array Max & Min(array=w135) -> (max value=w134:dbl)  [unwired: 3 out]
  }
  n58 = Array Size(array="cluster centers") -> (size(s)=w56:i32)
  n59 = Array Subset(array=w2, index (col)=0 ("index"), length (col)=4 ("length")) -> (w41:dbl[][])  [unwired: 2 in]
  n60 = Array Subset(array=w2, index (col)=0 ("index"), length (col)=4 ("length")) -> (w37:dbl[][])  [unwired: 2 in]
  n61 = Add(x=2, y=w56) -> (x+y=w55:i32)
  n62 = for {
    tunnel: w41 -> [w140] mode=indexing
    tunnel: [w136] -> w40 mode=indexing
    n63 = Array Max & Min(array=w140) -> (max value=w139:dbl)  [unwired: 3 out]
    n64 = for {
      tunnel: w140 -> [w168] mode=indexing
      tunnel: w139 -> [w167]
      tunnel: [w164] -> w137 mode=indexing if=w166
      i -> [w165]
      n65 = Equal?(x=w168, y=w167) -> (x = y?=w166:bool)
      n66 = Increment(x=w165) -> (x+1=w164:i32)
    }
    n67 = Array Size(array=w137) -> (size(s)=w138:i32)
    n68 = case shown="3" w138 {
      tunnel: w137 -> [_ w143 w147 w158]
      tunnel: [11 w142 w145 w157] -> w136
      frame 0, Default {
      }
      frame 1 {
        n69 = Index Array(array=w143) -> (element=w142:i32)  [unwired: 1 in]
      }
      frame 2 {
        n70 = for {
          tunnel: i32[][] [[1, 2], [2, 3], [3, 4], [1, 4], [1, 3], [2, 4]] -> [w153] mode=indexing
          tunnel: w147 -> [w152]
          tunnel: [w150] -> w144
          i -> [w150]
          stop <- w149 stop-if-true
          n71 = Equal?(x=w152, y=w153) -> (x = y?=w151:bool[])
          n72 = And Array Elements(Boolean array=w151) -> (logical AND=w149:bool)
        }
        n73 = Index Array(array=i32[] [7, 6, 8, 5, 9, 10], index=w144) -> (element=w145:i32)
      }
      frame 3 {
        n74 = for {
          tunnel: i32[][] [[1, 2, 3], [2, 3, 4], [1, 3, 4], [1, 2, 4]] -> [w163] mode=indexing
          tunnel: w158 -> [w162]
          tunnel: [w160] -> w156
          i -> [w160]
          stop <- w159 stop-if-true
          n75 = Equal?(x=w162, y=w163) -> (x = y?=w161:bool[])
          n76 = And Array Elements(Boolean array=w161) -> (logical AND=w159:bool)
        }
        n77 = Index Array(array=i32[] [9, 10, 9, 10], index=w156) -> (element=w157:i32)
      }
    }
  }
  n78 = for {
    tunnel: w37 -> [w212] mode=indexing
    tunnel: [w171] -> w38 mode=indexing
    tunnel: w32 -> [w208] mode=indexing
    tunnel: w30 -> [w183] mode=indexing
    tunnel: w28 -> [w173] mode=indexing
    tunnel: w23 -> [w182] mode=indexing
    tunnel: w19 -> [w177] mode=indexing
    (unwired) 11
    n79 = Array Max & Min(array=w208) -> (max value=w207:dbl, max index (indices)=w192:i32)  [unwired: 2 out]
    n80 = Array Max & Min(array=w177) -> (max value=w175:dbl)  [unwired: 3 out]
    n81 = Array Max & Min(array=w173) -> (max value=w176:dbl)  [unwired: 3 out]
    n82 = Array Max & Min(array=w182) -> (max value=w184:dbl, max index (indices)=w180:i32)  [unwired: 2 out]
    n83 = Equal?(x=w207, y=w183) -> (x = y?=w206:bool)
    n84 = for {
      tunnel: w208 -> [w227] mode=indexing
      tunnel: w207 -> [w226]
      tunnel: [w223] -> w205 mode=indexing if=w225
      i -> [w224]
      n85 = Equal?(x=w227, y=w226) -> (x = y?=w225:bool)
      n86 = Increment(x=w224) -> (x+1=w223:i32)
    }
    n87 = Build Array(w176, w175) -> ()  [unwired: 1 out]
    n88 = Array Max & Min(array=w212) -> (max value=w211:dbl)  [unwired: 3 out]
    n89 = Equal?(x=w184, y=w183) -> (x = y?=w185:bool)
    n90 = for {
      tunnel: w182 -> [w217] mode=indexing
      tunnel: w184 -> [w216]
      tunnel: [w213] -> w186 mode=indexing if=w215
      i -> [w214]
      n91 = Equal?(x=w217, y=w216) -> (x = y?=w215:bool)
      n92 = Increment(x=w214) -> (x+1=w213:i32)
    }
    n93 = Array Max & Min(array=w173) -> (max value=w196:dbl, max index (indices)=w191:i32)  [unwired: 2 out]
    n94 = for {
      tunnel: w212 -> [w255] mode=indexing
      tunnel: w211 -> [w254]
      tunnel: [w251] -> w209 mode=indexing if=w253
      i -> [w252]
      n95 = Equal?(x=w255, y=w254) -> (x = y?=w253:bool)
      n96 = Increment(x=w252) -> (x+1=w251:i32)
    }
    n97 = Array Size(array=w205) -> (size(s)=w204:i32)
    n98 = Equal?(x=w196, y=w183) -> (x = y?=w197:bool)
    n99 = Array Size(array=w186) -> (size(s)=w187:i32)
    n100 = for {
      tunnel: w173 -> [w222] mode=indexing
      tunnel: w196 -> [w221]
      tunnel: [w218] -> w198 mode=indexing if=w220
      i -> [w219]
      n101 = Equal?(x=w222, y=w221) -> (x = y?=w220:bool)
      n102 = Increment(x=w219) -> (x+1=w218:i32)
    }
    n103 = Equal?(x=w204, y=1) -> (x = y?=w202:bool)
    n104 = Equal?(x=w187, y=1) -> (x = y?=w189:bool)
    n105 = Array Size(array=w209) -> (size(s)=w210:i32)
    n106 = And(x=w206, y=w202) -> (x .and. y?=w195:bool)
    "x .and. y? 2" <- w195
    n107 = And(x=w185, y=w189) -> (x .and. y?=w179:bool)
    n108 = case shown="3" w210 {
      tunnel: w209 -> [_ w230 w234 w245]
      tunnel: [11 w229 w232 w244] -> w172
      frame 0, Default {
      }
      frame 1 {
        n109 = Index Array(array=w230) -> (element=w229:i32)  [unwired: 1 in]
      }
      frame 2 {
        n110 = for {
          tunnel: i32[][] [[1, 2], [2, 3], [3, 4], [1, 4], [1, 3], [2, 4]] -> [w240] mode=indexing
          tunnel: w234 -> [w239]
          tunnel: [w237] -> w231
          i -> [w237]
          stop <- w236 stop-if-true
          n111 = Equal?(x=w239, y=w240) -> (x = y?=w238:bool[])
          n112 = And Array Elements(Boolean array=w238) -> (logical AND=w236:bool)
        }
        n113 = Index Array(array=i32[] [7, 6, 8, 5, 9, 10], index=w231) -> (element=w232:i32)
      }
      frame 3 {
        n114 = for {
          tunnel: i32[][] [[1, 2, 3], [2, 3, 4], [1, 3, 4], [1, 2, 4]] -> [w250] mode=indexing
          tunnel: w245 -> [w249]
          tunnel: [w247] -> w243
          i -> [w247]
          stop <- w246 stop-if-true
          n115 = Equal?(x=w249, y=w250) -> (x = y?=w248:bool[])
          n116 = And Array Elements(Boolean array=w248) -> (logical AND=w246:bool)
        }
        n117 = Index Array(array=i32[] [9, 10, 9, 10], index=w243) -> (element=w244:i32)
      }
    }
    n118 = Array Size(array=w198) -> (size(s)=w199:i32)
    n119 = Increment(x=w192) -> (x+1=w193:i32)
    n120 = Equal?(x=w199, y=1) -> (x = y?=w201:bool)
    n121 = Add(x=w180, y=5) -> (x+y=w178:i32)
    n122 = And(x=w197, y=w201) -> (x .and. y?=w194:bool)
    "x .and. y?" <- w194
    n123 = Add(x=w191, y=9) -> (x+y=w174:i32)
    n124 = Select(t=w178, s=w179, f=w172) -> (s? t:f=w170:i32)
    n125 = Select(t=w174, s=w194, f=w170) -> (s? t:f=w169:i32)
    n126 = Select(t=w193, s=w195, f=w169) -> (s? t:f=w171:i32)
  }
  n127 = Initialize Array(0 ("index"), w55) -> (w54:i32[])
  n128 = Insert Into Array(array=w10, index (col)=8 ("disabled index (col)"), new element #1=w9, new element #2=w8) -> ()  [unwired: 1 in, 1 out]
  n129 = Number To Decimal String(number=w62) -> (decimal integer string=w3:string[])  [unwired: 1 in]
  "Assigned cluster (0) unassigned" <- w3
  n130 = Number To Decimal String(number=w46) -> (decimal integer string=w58:string[][])  [unwired: 1 in]
  n131 = Number To Fractional String(number=w2) -> (F-format string=w47:string[][])  [unwired: 3 in]
  n132 = Decimal String To Number(string=w3) -> (number=w60:i32[])  [unwired: 2 in, 1 out]
  n133 = Build Array (concatenate)("Patterns in", w58) -> (w61:string[][])
  n134 = Transpose 2D Array(2D array=w47) -> (transposed array=w48:string[][])
  n135 = for {
    tunnel: w60 -> [w258] mode=indexing
    shift-right: [w256] -> w59
    shift-left: w54 -> [w259]
    # "Count of elements assigned to \neash cluster"
    n136 = Index Array(array=w259, index=w258) -> (element=w260:i32)
    n137 = Increment(x=w260) -> (x+1=w257:i32)
    n138 = Replace Array Subset(array=w259, new element=w257, index=w258) -> (w256:i32[])
  }
  "Cluster element count" <- w59
  n139 = Transpose 2D Array(2D array=w61) -> (transposed array=w53:string[][])
  "patterns in, distance values" <- w53
  n140 = Index Array(array=w53, index (col)=0 ("disabled index (col)")) -> (element=w51:string[])  [unwired: 1 in]
  n141 = Build Array (concatenate)(w51, w3, w48) -> (w50:string[][])
  n142 = Transpose 2D Array(2D array=w50) -> (transposed array=→"appended array":string[][])
  n143 = Number To Decimal String(number=w40) -> (decimal integer string=→"Assigned cluster 2nd method":string[])  [unwired: 1 in]
  n144 = Number To Decimal String(number=w38) -> (decimal integer string=→"Assigned cluster 3rd method 2":string[])  [unwired: 1 in]
